vi "Main.vi"() -> ()   [LabVIEW 2020]
uses:
  controls/UI_Ref_Cluster.ctl
  controls/Car_wash_indicators.ctl
  Global variables/Elapsed_time.vi
  Global variables/Time_to_elapse.vi
  Global variables/Bad_position.vi
  Global variables/Delay_time.vi
  Global variables/Reset_timer.vi
  <vilib>/vision/driver/NI_Vision_Acquisition_Software.lvlib
  <vilib>/userDefined/High Color/IMAQdx.ctl
  <vilib>/vision/NI_Vision_Development_Module.lvlib
  <vilib>/drjdpowell/SQLite Library/SQL Connection/Connection.lvclass
  <vilib>/drjdpowell/SQLite Library/SQL Connection/Open (path).vi
  <vilib>/drjdpowell/SQLite Library/SQLite.lvlib
  <vilib>/drjdpowell/SQLite Library/SQL Connection/Execute SQL (No results).vi
  <vilib>/drjdpowell/SQLite Library/SQL Connection/Execute SQL.vi
  controls/Wash_options.ctl
panel:
  out "Result Set":string[][](table) caption="Result Set (from first statement with results)"
  in  "Show Database":bool
  out "SQL_Expression":string
  out "Exit_Panel":bool
  out "Image":T1(plugin-control)
  out "Read String":string
  out "License Plate":string
  in  "Array":i8[](array[numeric])=[0, 1, 2, 3, 4, 5, 6, 7]
  out "Info_for_driver":string
  in  "Car position slider":i8(slide)=1 scale=0.0..7.0
  in  "Start Button":bool
  out "Elapsed Time":dbl format="%.2f"
  in  "Stop Button":bool
  out "Car wash indicators":T2
  in  "Wash Options":T3
  out "Wash entry":bool
  # "Entry console"
  # "Car Wash Dispaly"
  # "Wash Entry"
  # "Wash Options"
  # "Car Wash Indicators"
  # "Car Wash Indicators"
  # "Elapsed Time"
  # "Start"
  # "Car position simulation"
  # "Pre-Soak\nH-P Wash\nL-P Wax\nSpot Free Rinse"
  # "Underbody Wash\nBug Remover"
  # "Tire Shine\nAir Dry"
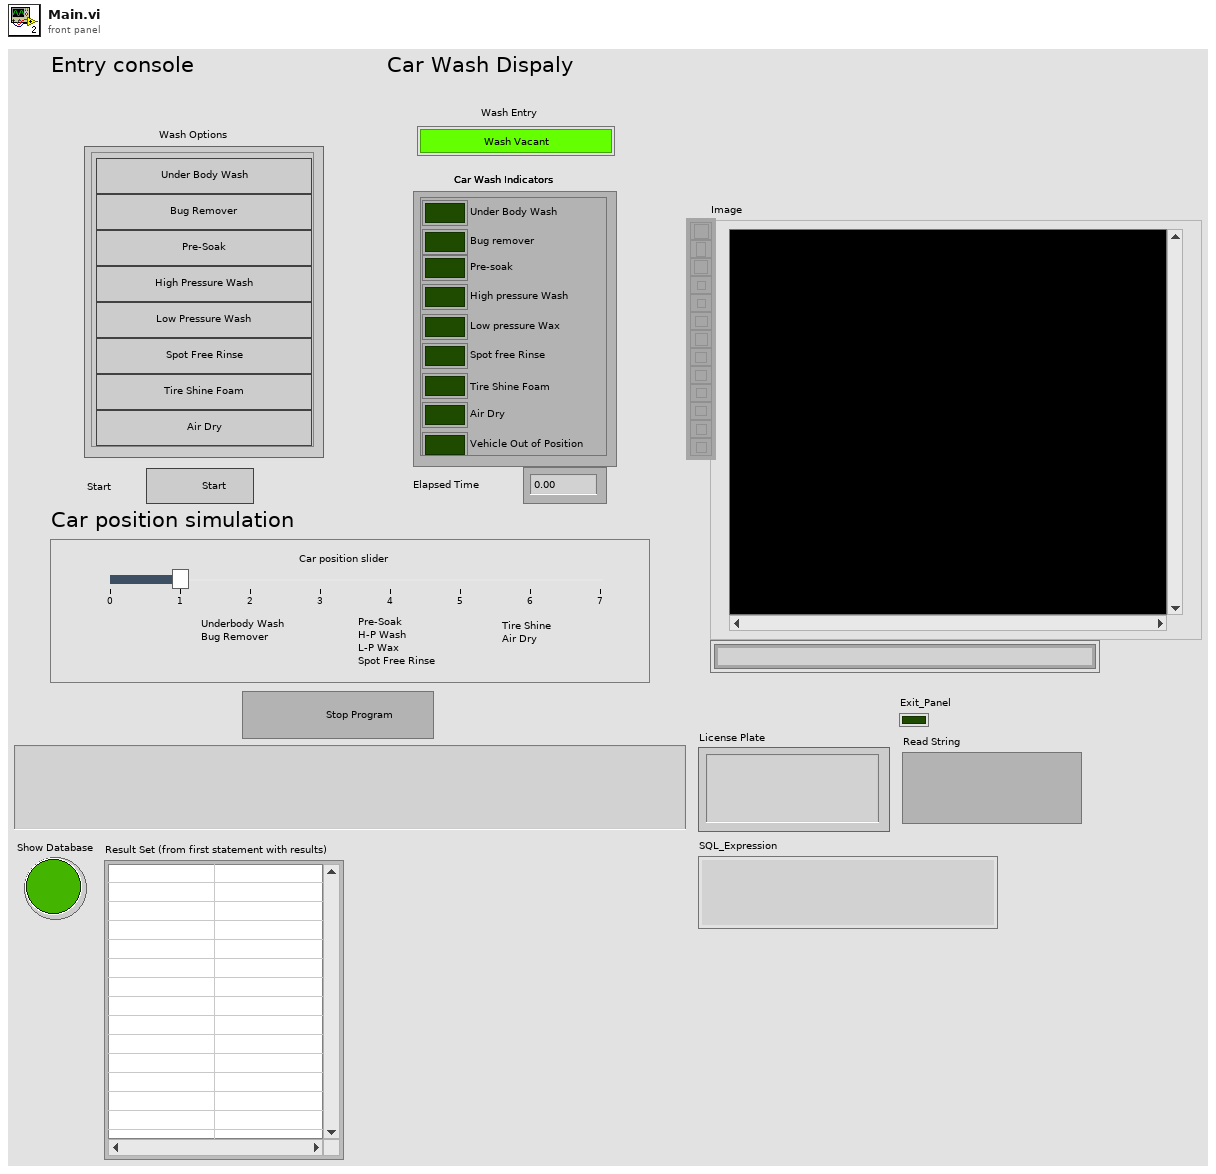
[diagram p1: front panel]
types:
  T1 = typedef "IMAQ Image.ctl" = refnum<image>
  T2 = typedef "Car_wash_indicators.ctl" = cluster{"Under Body Wash":bool, "Bug remover":bool, "Pre-soak":bool, "High pressure Wash":bool, "Low pressure Wax":bool, "Spot free Rinse ":bool, "Tire Shine Foam ":bool, "Air Dry ":bool, "Vehicle Out of Position":bool}
  T3 = typedef "Wash_options.ctl" = cluster{"Under body wash":bool, "Bug remover":bool, "Pre-soak":bool, "High pressure":bool, "Low pressure":bool, "Spot free Rinse":bool, "Tire Shine Foam":bool, "Air Dry":bool}
  T4 = typedef "IMAQ Rectangle" = cluster{"Left":i32, "Top":i32, "Right":i32, "Bottom":i32, "Rotation":dbl}
  T5 = typedef "IMAQdx.ctl" = refnum<k21>
  T6 = typedef "IMAQ OCR Session.ctl" = refnum<k1>
  T7 = enum32{"Invalid", "Standard", "Closed", "Hidden", "Minimized", "Maximized"}
  T8 = enum32{"invalid app kind", "Development System", "Run Time System", "Student Edition", "Embedded LabVIEW", "Evaluation", "Custom"}
  T9 = enum8{"Enabled", "Disabled", "Disabled and Grayed Out"}
  T10 = typedef "UI_Ref_Cluster.ctl" = cluster{"Stop Button Ref":refnum<vi>, "Start Button Ref":refnum<vi>, "Elapsed Time Ref":refnum<vi>, "Car wash indicators Ref":refnum<vi>, "Wash Options Ref":refnum<vi>, "Wash entry Ref":refnum<vi>, "Car position slider Ref":refnum<vi>, "Info_for_driver Ref":refnum<vi>, "Array Ref":refnum<vi>, "License Plate Ref":refnum<vi>}
  T11 = cluster{"Core":cluster{"Current VI Reference":refnum<vi>, "Close Panel on Exit?":bool}, "UI_Cluster_Out":T10}
  T12 = cluster{"Current VI Reference":refnum<vi>, "Close Panel on Exit?":bool}
  T13 = typedef "ROI Descriptor" = cluster{"Global Rectangle":i32[], "Contours":cluster{"ID":enum32{"External", "Internal"}, "Type":u32, "Coordinates":i32[]}[]}
  T14 = cluster{"Global Rectangle":i32[], "Contours":cluster{"ID":enum32{"External", "Internal"}, "Type":u32, "Coordinates":i32[]}[]}
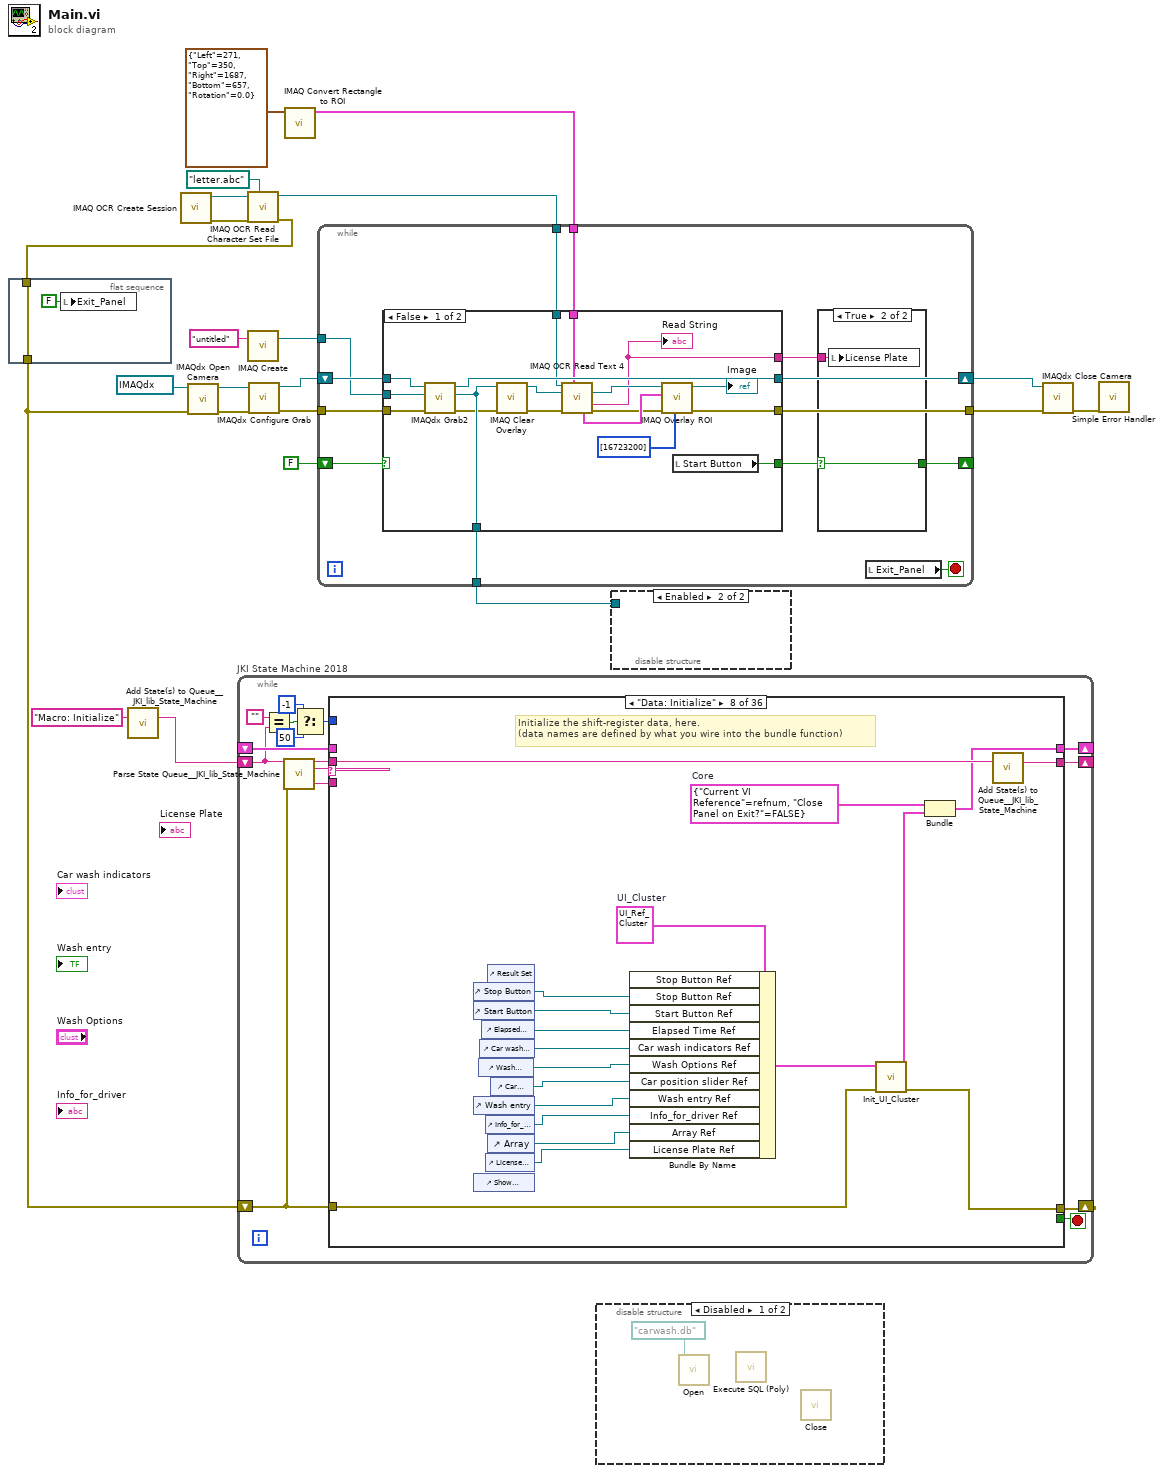
[diagram p0: block diagram]
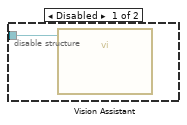
[diagram p2: hidden frame]
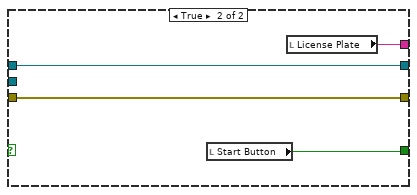
[diagram p5: hidden frame]
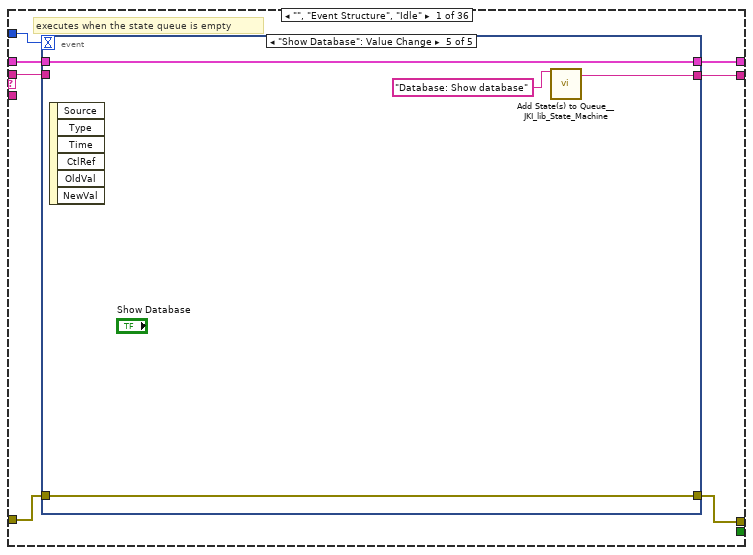
[diagram p6: hidden frame]
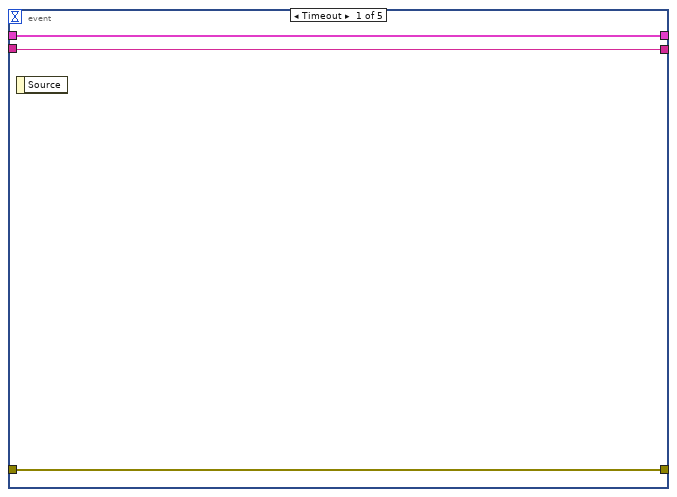
[diagram p7: hidden frame]
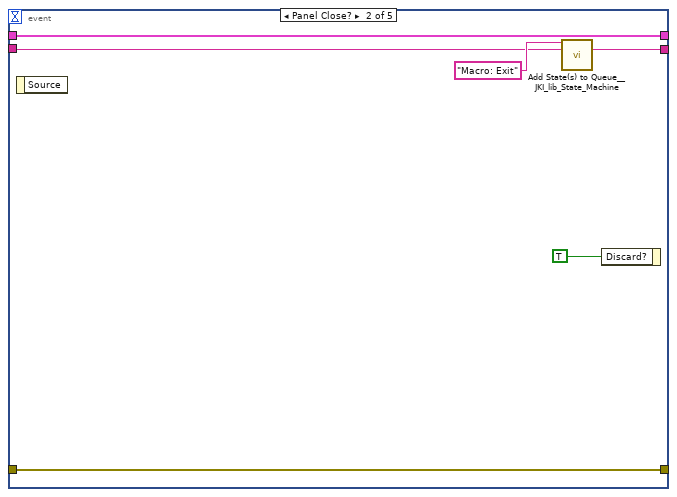
[diagram p8: hidden frame]
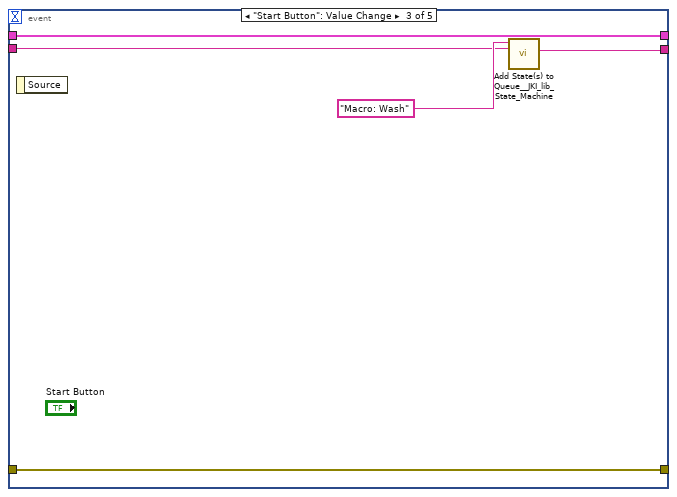
[diagram p9: hidden frame]
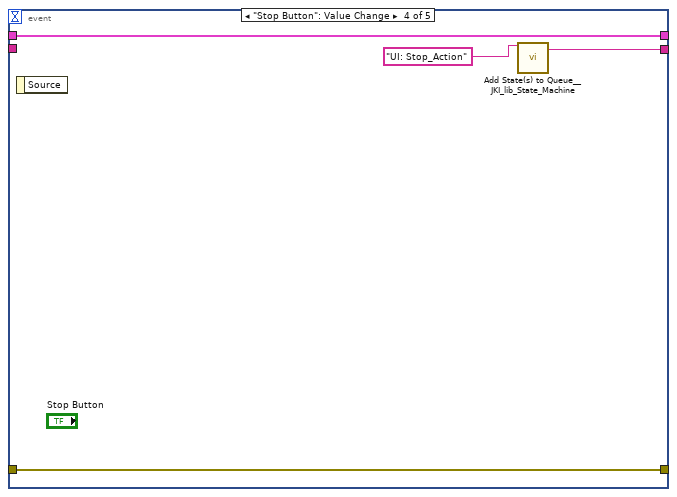
[diagram p10: hidden frame]
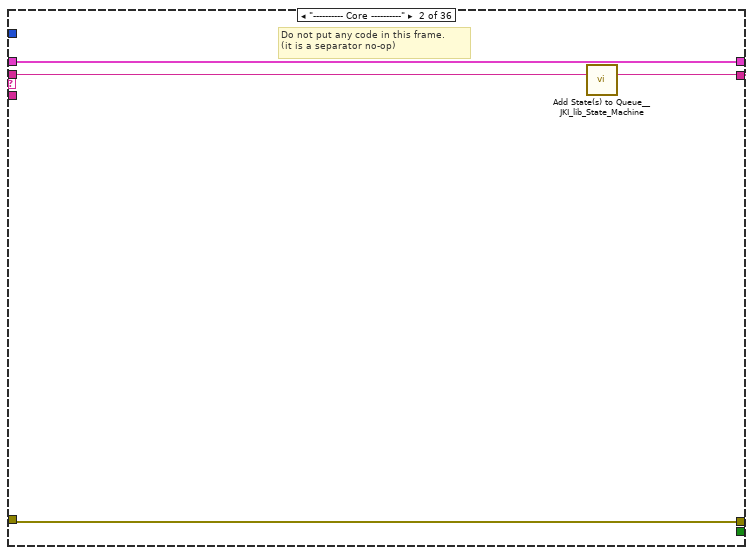
[diagram p11: hidden frame]
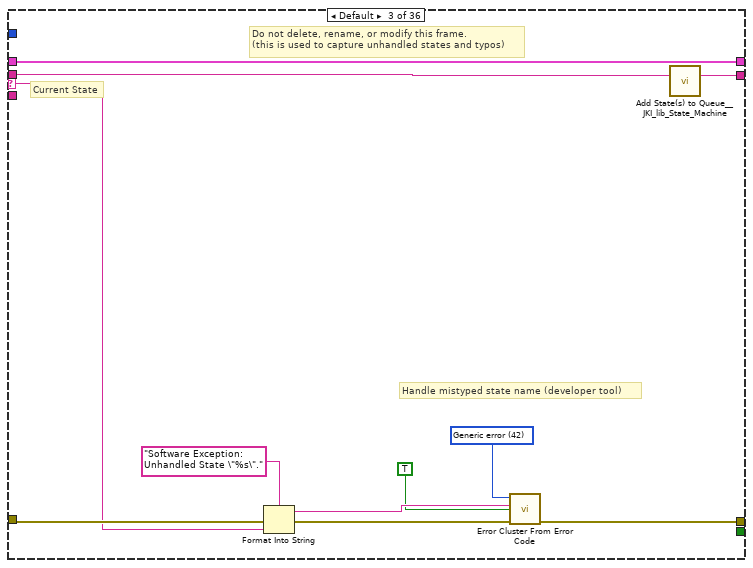
[diagram p12: hidden frame]
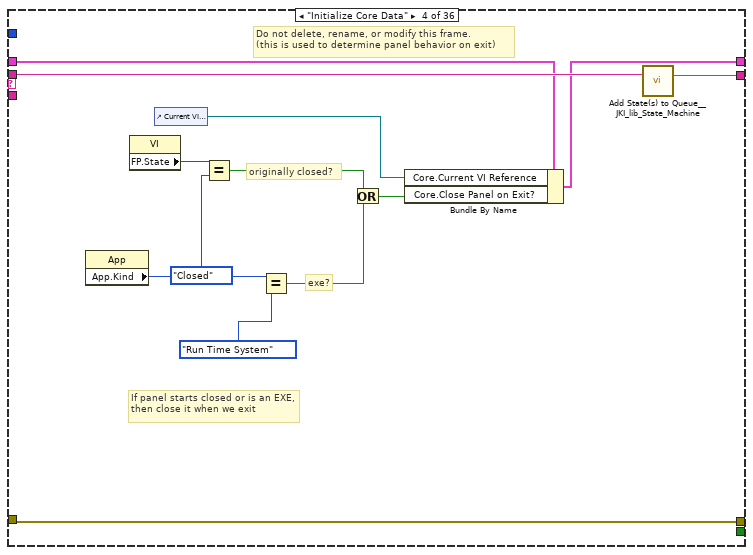
[diagram p13: hidden frame]
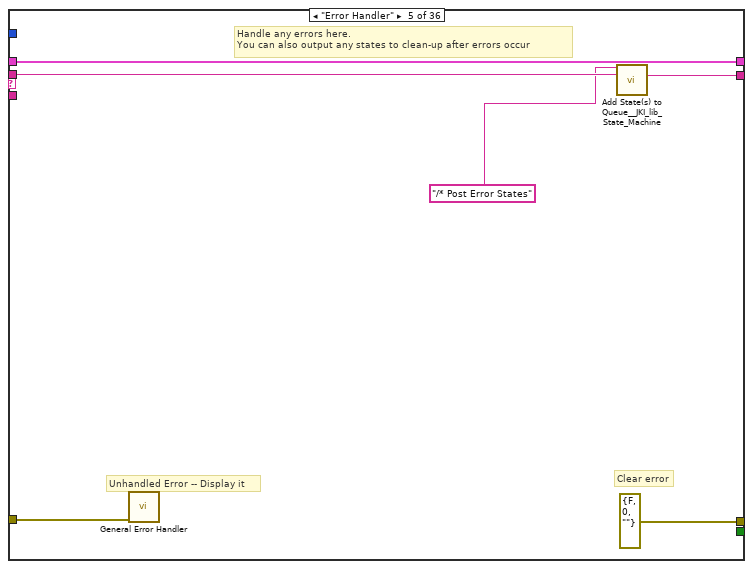
[diagram p14: hidden frame]
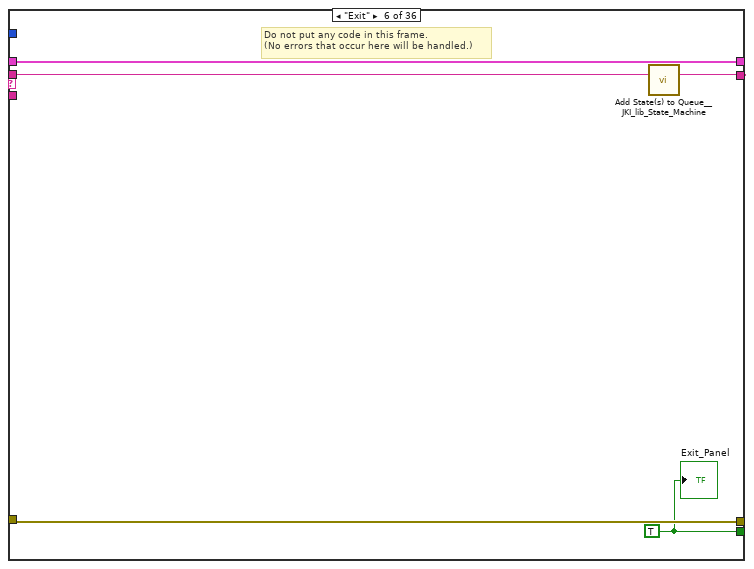
[diagram p15: hidden frame]
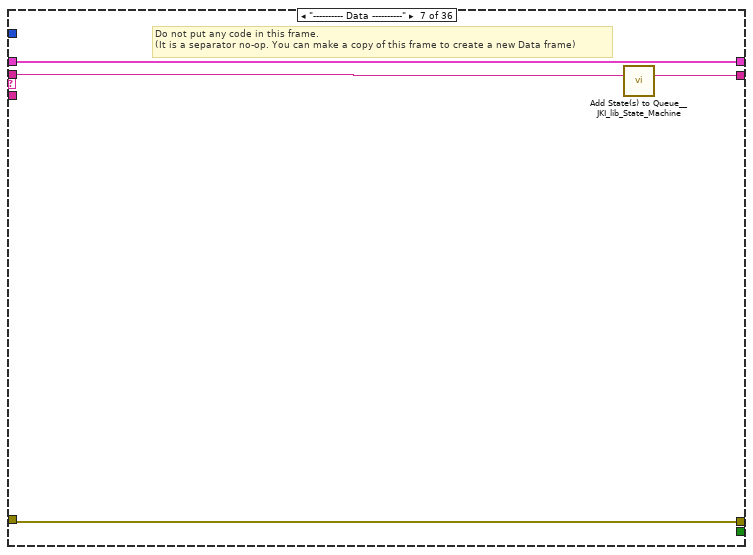
[diagram p16: hidden frame]
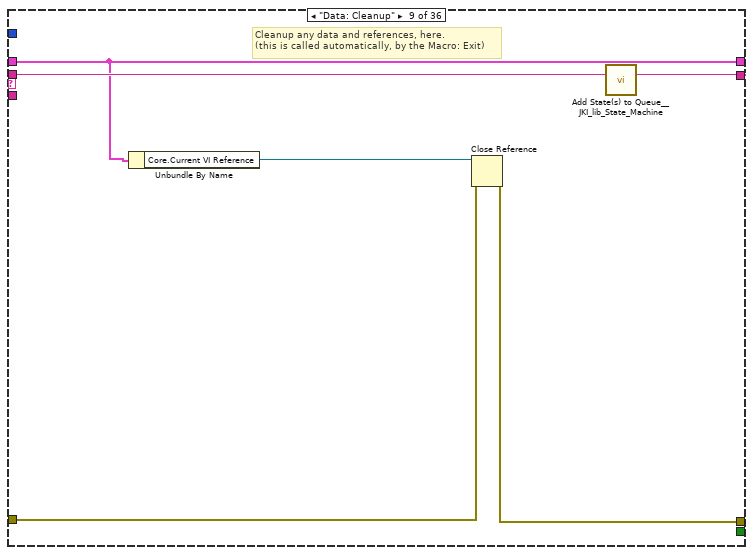
[diagram p17: hidden frame]
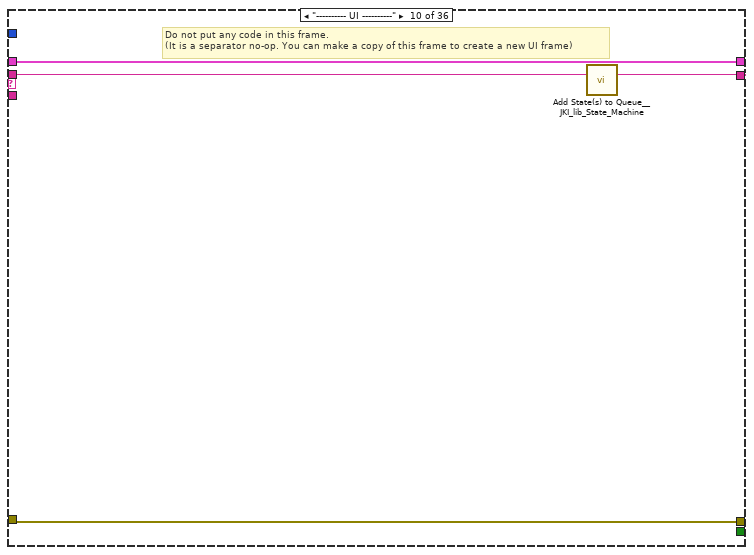
[diagram p18: hidden frame]
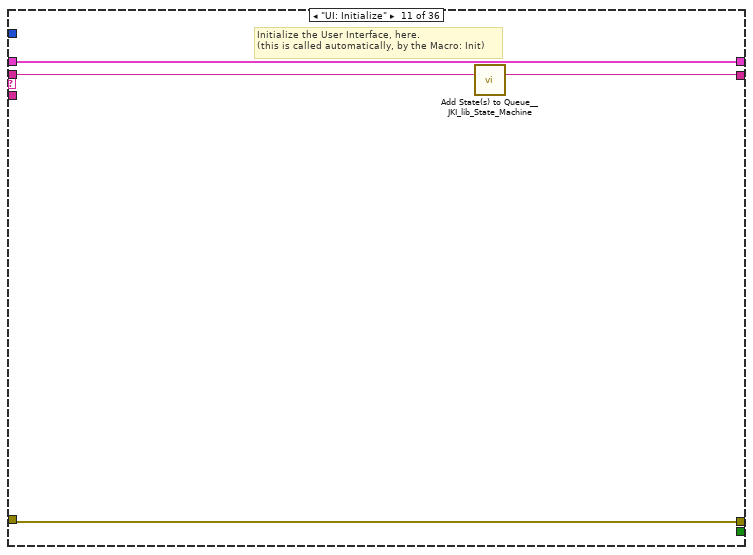
[diagram p19: hidden frame]
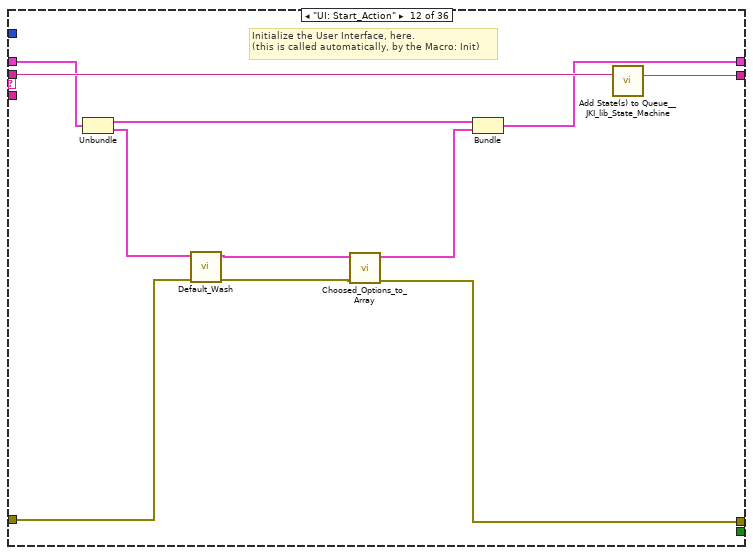
[diagram p20: hidden frame]
diagram:
  n1 = flat-sequence {
    tunnel: w4 -> [w23]
    tunnel: [w23] -> w3
    frame #0 {
      n2 = local write "Exit_Panel"(FALSE) -> ()
    }
  }
  n3 = call <vilib>:"Add State(s) to Queue__JKI_lib_State_Machine.vi"("State(s) in (\"\")"="Macro: Initialize") -> ("States Out"=w22:string)  [unwired: 14 in]
  n4 = call "IMAQ OCR Create Session"() -> ("error out"=w16:errorcluster, "IMAQ OCR Session"=w15:T6)  [unwired: 10 in]
  n5 = call <vilib>:"IMAQdx Open Camera.vi"("error in"=w3, "Session In"=T5 "cam0") -> ("error out"=w7:errorcluster, "Session Out"=w8:T5)  [unwired: 8 in]
  n6 = while "JKI State Machine 2018" {
    shift-right: [w34] -> _
    shift-left: _ -> [w33]
    shift-right: [w36] -> _
    shift-left: w3 -> [w32]
    shift-right: [w35] -> _
    shift-left: w22 -> [w30]
    stop <- w25 stop-if-true
    n7 = Equal?(x="", y=w30) -> (x = y?=w29:bool)
    n8 = call <vilib>:"Parse State Queue__JKI_lib_State_Machine.vi"("State Queue"=w30, "Error In (no error)"=w32) -> ("Remaining States"=w38:string, "Current State"=w39:string, "Arguments"=w37:string)  [unwired: 11 in]
    n9 = Select(t=-1, s=w29, f=50) -> (s? t:f=w28:i32)
    n10 = case shown="\"Data: Initialize\"" w39 {
      selector: w39 -> [_ _ w73 _ _ _ _ _ _ _ _ _ _ _ _ _ _ _ _ _ _ _ _ _ _ _ _ _ _ _ _ _ _ _ _ _]
      tunnel: w38 -> [w41 w72 w77 w96 w102 w107 w111 w130 w136 w140 w144 w155 w164 w170 w181 w245 w250 w255 w265 w269 w273 w303 w306 w339 w379 w419 w459 w499 w539 w579 w619 w658 w664 w671 w684 w689]
      tunnel: w37 -> [_ _ _ _ _ _ _ _ _ _ _ _ _ w166 w176 _ _ _ _ _ _ w300 _ _ _ _ _ _ _ _ _ _ _ _ _ _]
      tunnel: w33 -> [w46 w69 w75 w85 w100 w105 w108 _ w132 w137 w142 w153 w162 w168 w175 w242 w247 w252 w257 w266 w276 w295 w311 w334 w376 w413 w451 w491 w531 w571 w611 w655 w659 w672 w681 w687]
      tunnel: [w45 w70 w79 w94 errorcluster {"status"=FALSE, "code"=0, "source"=""} ("error out") w104 w109 w118 w133 w138 w141 w147 w159 w167 w178 w243 w248 w253 w263 w267 w272 w301 w312 w337 w377 w410 w457 w497 w537 w577 w617 w656 w662 w669 w674 w686] -> w36
      tunnel: w32 -> [w44 w70 w78 w94 w99 w104 w109 w119 w134 w138 w141 w149 w160 w165 w179 w243 w248 w253 w263 w267 w272 w301 w312 w337 w377 w410 w457 w497 w537 w577 w617 w656 w662 w669 w674 w686]
      tunnel: [w40 w71 w76 w95 w101 w106 w110 w129 w135 w139 w143 w154 w163 w169 w180 w244 w249 w254 w264 w268 w277 w302 w305 w338 w378 w418 w458 w498 w538 w578 w618 w657 w663 w670 w683 w688] -> w35
      tunnel: [_ _ _ _ _ w103 _ _ _ _ _ _ _ _ _ _ _ _ _ _ _ _ _ _ _ _ _ _ _ _ _ _ _ _ _ _] -> w25
      tunnel: [w43 w69 w75 w84 w100 w105 w108 w121 w132 w137 w142 w151 w156 w168 w175 w242 w247 w252 w257 w266 w276 w295 w311 w334 w376 w413 w451 w491 w531 w571 w611 w655 w659 w672 w681 w687] -> w34
      tunnel: w28 -> [w42 _ _ _ _ _ _ _ _ _ _ _ _ _ _ _ _ _ _ _ _ _ _ _ _ _ _ _ _ _ _ _ _ _ _ _]
      frame "", "Event Structure", "Idle" {
        # "executes when the state queue is empty"
        n11 = event shown="[4] \"Show Database\": Value Change" {
          selector: _ -> [_ _ _ _ _]
          dyn-events: _ -> [_ _ _ _ _]
          timeout: w42 -> [_ _ _ _ _]
          tunnel: w46 -> [w48 w54 w60 w64 w68]
          tunnel: [w49 w55 w58 w62 w66] -> w45
          tunnel: w44 -> [w49 w55 w58 w62 w66]
          tunnel: [w48 w54 w60 w64 w68] -> w43
          tunnel: [w47 w51 w56 w61 w65] -> w40
          tunnel: w41 -> [w47 w50 w57 _ _]
          event Timeout {
            n12 = event-data() -> ()  [unwired: 1 in, 1 out]
          }
          event Panel Close? {
            n13 = event-data() -> ()  [unwired: 1 in, 1 out]
            n14 = call <vilib>:"Add State(s) to Queue__JKI_lib_State_Machine.vi"("State(s) in Front (\"\")"="Macro: Exit", "State(s) in (\"\")"=w50) -> ("States Out"=w51:string)  [unwired: 13 in]
            n15 = event-data("Discard?"=TRUE) -> ()  [unwired: 1 in, 1 out]
          }
          event "Start Button": Value Change {
            n16 = event-data() -> ()  [unwired: 1 in, 1 out]
            n17 = call <vilib>:"Add State(s) to Queue__JKI_lib_State_Machine.vi"("State(s) in Front (\"\")"="Macro: Wash", "State(s) in (\"\")"=w57) -> ("States Out"=w56:string)  [unwired: 13 in]
          }
          event "Stop Button": Value Change {
            n18 = event-data() -> ()  [unwired: 1 in, 1 out]
            n19 = call <vilib>:"Add State(s) to Queue__JKI_lib_State_Machine.vi"("State(s) in Front (\"\")"="UI: Stop_Action") -> ("States Out"=w61:string)  [unwired: 14 in]
          }
          event "Show Database": Value Change {
            n20 = event-data() -> ()  [unwired: 1 in, 6 out]
            n21 = call <vilib>:"Add State(s) to Queue__JKI_lib_State_Machine.vi"("State(s) in Front (\"\")"="Database: Show database") -> ("States Out"=w65:string)  [unwired: 14 in]
          }
        }
      }
      frame "---------- Core ----------" {
        # "Do not put any code in this frame.\n(it is a separator no-op)"
        n22 = call <vilib>:"Add State(s) to Queue__JKI_lib_State_Machine.vi"("State(s) in (\"\")"=w72) -> ("States Out"=w71:string)  [unwired: 14 in]
      }
      frame Default {
        w82 = 42 items=["No error", "Argument error", "Memory is full", "Out of zone", "End of file", "File already open", "Generic file I/O error", "File not found", "File permission error", "Disk is full", "Duplicate path", "Too many files open", "System feature not enabled", "Resource file not found", "Cannot add resource", "Resource not found", "Image not found", "Image memory error", "Pen does not exist", "Config type invalid", "Config token not found", "Config parse error", "Config memory error", "Bad external code format", "Bad external code offset", "External code not present", "Null window", "Destroy window error", "Null menu", "Print aborted", "Bad print record", "Print driver error", "Windows error during printing", "Memory error during printing", "Print dialog error", "Generic print error", "Invalid device refnum", "Device not found", "Device parameter error", "Device unit error", "Cannot open device", "Device call aborted", "Generic error", "Cancelled by user", "Object ID too low", "Object ID too high", "Object not in heap", "Unknown heap", "Unknown object (invalid DefProc)", "Unknown object (DefProc not in table)", "Message out of range", "Invalid (null) method", "Unknown message", "Manager call not supported", "Bad address", "Network operation in progress", "Network operation timed out", "Connection is busy", "Network attribute not supported", "Network error", "Address in use", "System out of memory", "Connection aborted", "Connection refused", "Not connected", "Already connected", "Connection closed", "Initialization error (interapplication manager)", "Bad occurrence", "Wait on unbound occurrence handler", "Occurrence queue overflow", "Datalog type conflict", "Unused", "Unrecognized type (interapplication manager)", "Memory corrupt", "Failed to make temporary DLL", "Old CIN version", "Drag socket not found", "Failed to load drop-object", "Failed to register OLE object", "Failed to release OLE object", "Format specifier type mismatch", "Unknown format specifier", "Too few format specifiers", "Too many format specifiers", "Scan failed", "Newer CIN version", "Error converting to variant", "Runtime menu error", "Password tampered", "Variant attribute not found", "Incompatible variant data type", "Event data is not available", "Event Store is not present", "Occurrence is not found", "Event Queue is not created", "Event info is not available", "Refnum passed is NULL", "Error retrieving Class GUID", "Error retrieving CoClass GUID", "Error retrieving TypeLib GUID.", "Bad built application magic bytes.", "Specific driver is different from the specific driver associated with the Logical Name.", "There is no session opened to the class driver.", "Max Error", "MAX - Error with config objects", "MAX - Error loading configuration", "MAX - Group not supported"]
        # "Current State"
        # "Do not delete, rename, or modify this frame.\n(this is used to capture unhandled states and typos)"
        # "Handle mistyped state name (developer tool)"
        n23 = Format Into String(format string="Software Exception: Unhandled State \"%s\"." ("message"), error in=w78, w73) -> (resulting string=w81:string, error out=w80:errorcluster)  [unwired: 1 in]
        n24 = call <vilib>:"Error Cluster From Error Code.vi"("show call chain? (False)"=TRUE, "error in (no error)"=w80, "error message (\"\")"=w81, "error code (0)"=w82) -> ("error out"=w79:errorcluster)  [unwired: 5 in]
        n25 = call <vilib>:"Add State(s) to Queue__JKI_lib_State_Machine.vi"("State(s) in (\"\")"=w77) -> ("States Out"=w76:string)  [unwired: 14 in]
      }
      frame "Initialize Core Data" {
        # "Do not delete, rename, or modify this frame.\n(this is used to determine panel behavior on exit)"
        # "originally closed?"
        # "exe?"
        # "If panel starts closed or is an EXE, then close it when we exit"
        n26 = property class="App"() -> ("App.Kind"=w93:T8)  [unwired: 2 in, 2 out]
        n27 = property class="VI"() -> ("FP.State"=w88:T7)  [unwired: 2 in, 2 out]
        n28 = control-ref of="Current VI Reference"() -> (w89:refnum<vi>)
        n29 = Equal?(x=w88, y=T7."Closed" ("Front Panel Window:State")) -> (x = y?=w86:bool)
        n30 = Equal?(x=w93, y=T8."Run Time System" ("Application:Kind")) -> (x = y?=w91:bool)
        n31 = Or(x=w86, y=w91) -> (x .or. y?=w90:bool)
        n32 = Bundle By Name(cluster=w85, "Core.Current VI Reference"=w89, "Core.Close Panel on Exit?"=w90) -> (w84:T11)
        n33 = call <vilib>:"Add State(s) to Queue__JKI_lib_State_Machine.vi"("State(s) in (\"\")"=w96) -> ("States Out"=w95:string)  [unwired: 14 in]
      }
      frame "Error Handler" {
        # "Unhandled Error -- Display it"
        # "Handle any errors here.\nYou can also output any states to clean-up after errors occur"
        # "Clear error"
        n34 = call <vilib>:"General Error Handler.vi"("error in (no error)"=w99) -> ()  [unwired: 10 in, 5 out]
        n35 = call <vilib>:"Add State(s) to Queue__JKI_lib_State_Machine.vi"("State(s) in Front (\"\")"="/* Post Error States", "State(s) in (\"\")"=w102) -> ("States Out"=w101:string)  [unwired: 13 in]
      }
      frame "Exit" {
        w103 = TRUE
        # "Do not put any code in this frame.\n(No errors that occur here will be handled.)"
        n36 = call <vilib>:"Add State(s) to Queue__JKI_lib_State_Machine.vi"("State(s) in (\"\")"=w107) -> ("States Out"=w106:string)  [unwired: 14 in]
        "Exit_Panel" <- w103
      }
      frame "---------- Data ----------" {
        # "Do not put any code in this frame.\n(It is a separator no-op. You can make a copy of this frame to create a new Data frame)"
        n37 = call <vilib>:"Add State(s) to Queue__JKI_lib_State_Machine.vi"("State(s) in (\"\")"=w111) -> ("States Out"=w110:string)  [unwired: 14 in]
      }
      frame "Data: Initialize" {
        w113 = T10 {"Stop Button Ref"=refnum, "Start Button Ref"=refnum, "Elapsed Time Ref"=refnum, "Car wash indicators Ref"=refnum, "Wash Options Ref"=refnum, "Wash entry Ref"=refnum, "Car position slider Ref"=refnum, "Info_for_driver Ref"=refnum, "Array Ref"=refnum, "License Plate Ref"=refnum}  # UI_Cluster
        w128 = T12 {"Current VI Reference"=refnum, "Close Panel on Exit?"=FALSE}  # Core
        # "Initialize the shift-register data, here.\n(data names are defined by what you wire into the bundle function)"
        n38 = control-ref of="Stop Button"() -> (w126:refnum<vi>)
        n39 = control-ref of="Start Button"() -> (w125:refnum<vi>)
        n40 = control-ref of="Wash entry"() -> (w122:refnum<vi>)
        n41 = control-ref of="Show Database"() -> ()  [unwired: 1 out]
        n42 = control-ref of="Wash Options"() -> (w117:refnum<vi>)
        n43 = control-ref of="Car wash indicators"() -> (w123:refnum<vi>)
        n44 = control-ref of="Elapsed Time"() -> (w124:refnum<vi>)
        n45 = control-ref of="Info_for_driver"() -> (w115:refnum<vi>)
        n46 = control-ref of="License Plate"() -> (w112:refnum<vi>)
        n47 = control-ref of="Result Set"() -> ()  [unwired: 1 out]
        n48 = control-ref of="Array"() -> (w114:refnum<vi>)
        n49 = control-ref of="Car position slider"() -> (w116:refnum<vi>)
        n50 = Bundle By Name "Bundle By Name"(cluster=w113, "Stop Button Ref"=w126, "Start Button Ref"=w125, "Elapsed Time Ref"=w124, "Car wash indicators Ref"=w123, "Wash Options Ref"=w117, "Car position slider Ref"=w116, "Wash entry Ref"=w122, "Info_for_driver Ref"=w115, "Array Ref"=w114, "License Plate Ref"=w112) -> (w127:T10)  [unwired: 1 in]
        n51 = call "Init_UI_Cluster.vi"("UI_Cluster_In"=w127, "error in"=w119) -> ("UI_Cluster_Out"=w120:T10, "error out"=w118:errorcluster)  [unwired: 7 in]
        n52 = Bundle("Core"=w128, "UI_Cluster_Out"=w120) -> (w121:T11)  [unwired: 1 in]
        n53 = call <vilib>:"Add State(s) to Queue__JKI_lib_State_Machine.vi"("State(s) in (\"\")"=w130) -> ("States Out"=w129:string)  [unwired: 14 in]
      }
      frame "Data: Cleanup" {
        # "Cleanup any data and references, here.\n(this is called automatically, by the Macro: Exit)"
        n54 = Unbundle By Name(w132) -> ("Core.Current VI Reference"=w131:refnum<vi>)
        n55 = Close Reference(reference=w131, error in (no error)=w134) -> (error out=w133:errorcluster)
        n56 = call <vilib>:"Add State(s) to Queue__JKI_lib_State_Machine.vi"("State(s) in (\"\")"=w136) -> ("States Out"=w135:string)  [unwired: 14 in]
      }
      frame "---------- UI ----------" {
        # "Do not put any code in this frame.\n(It is a separator no-op. You can make a copy of this frame to create a new UI frame)"
        n57 = call <vilib>:"Add State(s) to Queue__JKI_lib_State_Machine.vi"("State(s) in (\"\")"=w140) -> ("States Out"=w139:string)  [unwired: 14 in]
      }
      frame "UI: Initialize" {
        # "Initialize the User Interface, here.\n(this is called automatically, by the Macro: Init)"
        n58 = call <vilib>:"Add State(s) to Queue__JKI_lib_State_Machine.vi"("State(s) in (\"\")"=w144) -> ("States Out"=w143:string)  [unwired: 14 in]
      }
      frame "UI: Start_Action" {
        # "Initialize the User Interface, here.\n(this is called automatically, by the Macro: Init)"
        n59 = Unbundle(w153) -> ("Core"=w152:T12, "UI_Cluster_Out"=w150:T10)
        n60 = call "Default_Wash.vi"("UI_Cluster_In"=w150, "error in"=w149) -> ("UI_Cluster_Out"=w145:T10, "error out"=w148:errorcluster)  [unwired: 7 in]
        n61 = call "Choosed_Options_to_Array.vi"("error in (no error)"=w148, "UI_Cluster_In"=w145) -> ("error out"=w147:errorcluster, "UI_Cluster_Out"=w146:T10)  [unwired: 8 in]
        n62 = Bundle("Core"=w152, "UI_Cluster_Out"=w146) -> (w151:T11)  [unwired: 1 in]
        n63 = call <vilib>:"Add State(s) to Queue__JKI_lib_State_Machine.vi"("State(s) in (\"\")"=w155) -> ("States Out"=w154:string)  [unwired: 14 in]
      }
      frame "UI: Stop_Action" {
        n64 = Unbundle(w162) -> ("Core"=w158:T12, "UI_Cluster_Out"=w161:T10)
        n65 = call "Stop_UI_Cluster.vi"("UI_Cluster_In"=w161, "error in"=w160) -> ("UI_Cluster_Out"=w157:T10, "error out"=w159:errorcluster)  [unwired: 7 in]
        n66 = Bundle("Core"=w158, "UI_Cluster_Out"=w157) -> (w156:T11)  [unwired: 1 in]
        n67 = call <vilib>:"Add State(s) to Queue__JKI_lib_State_Machine.vi"("State(s) in (\"\")"=w164) -> ("States Out"=w163:string)  [unwired: 14 in]
      }
      frame "UI: Cursor Set" {
        # "Argument"
        # "Set and Unset Cursor Busy.\n(Usage: \"UI: Cursor Set >> Busy|Idle\")"
        n68 = case shown="\"Idle\", Default" w166 {
          tunnel: w165 -> [w172 w174]
          tunnel: [w171 w173] -> w167
          frame "Idle", Default {
            n69 = call <vilib>:"Unset Busy.vi"("error in (no error)"=w172) -> ("error out"=w171:errorcluster)  [unwired: 10 in]
          }
          frame "Busy" {
            n70 = call <vilib>:"Set Busy.vi"("error in (no error)"=w174) -> ("error out"=w173:errorcluster)  [unwired: 9 in, 1 out]
          }
        }
        n71 = call <vilib>:"Add State(s) to Queue__JKI_lib_State_Machine.vi"("State(s) in (\"\")"=w170) -> ("States Out"=w169:string)  [unwired: 14 in]
      }
      frame "UI: Front Panel State" {
        # "Argument"
        # "Set Front Panel Open or Closed\n(Usage: \"UI: Front Panel State >> Open|Close\")"
        n72 = Unbundle By Name(w175) -> ("Core.Current VI Reference"=w177:refnum<vi>)
        n73 = case shown="\"Minimize\", \"Minimized\"" w176 {
          tunnel: w179 -> [w187 w200 w211 w223 w235]
          tunnel: [w188 w201 w212 w224 w236] -> w178
          tunnel: w177 -> [_ _ _ _ _]
          frame "Open", "Standard", Default {
            w182 = T7."Standard" ("State")
            n74 = property class="VI"(error in=w187) -> (reference out=w185:refnum<vi>, error out=w186:errorcluster, "FP.State"=w184:T7)  [unwired: 1 in]
            n75 = Not Equal?(x=w184, y=w182) -> (x != y?=w183:bool)
            n76 = case shown="True" w183 {
              tunnel: [w192 w194] -> w188
              tunnel: w186 -> [w191 w194]
              tunnel: w185 -> [w190 _]
              tunnel: w182 -> [w189 _]
              frame True {
                n77 = invoke class="VI" method="FP.Open"(reference=w190, error in=w191, "Activate"=TRUE, "State"=w189) -> (error out=w192:errorcluster)  [unwired: 1 in, 4 out]
              }
              frame False {
              }
            }
          }
          frame "Close", "Closed" {
            n78 = property class="VI"(error in=w200) -> (reference out=w198:refnum<vi>, error out=w199:errorcluster, "FP.State"=w196:T7)  [unwired: 1 in]
            n79 = Not Equal?(x=w196, y=T7."Closed" ("Front Panel Window:State")) -> (x != y?=w195:bool)
            n80 = case shown="True" w195 {
              tunnel: [w202 w205] -> w201
              tunnel: w199 -> [w202 w204]
              tunnel: w198 -> [_ w203]
              frame False {
              }
              frame True {
                n81 = invoke class="VI" method="FP.Close"(reference=w203, error in=w204) -> (error out=w205:errorcluster)  [unwired: 1 in, 2 out]
              }
            }
          }
          frame "Hidden", "Hide" {
            w206 = T7."Hidden" ("State")
            n82 = property class="VI"(error in=w211) -> (reference out=w209:refnum<vi>, error out=w210:errorcluster, "FP.State"=w208:T7)  [unwired: 1 in]
            n83 = Not Equal?(x=w208, y=w206) -> (x != y?=w207:bool)
            n84 = case shown="True" w207 {
              tunnel: [w216 w217] -> w212
              tunnel: w210 -> [w215 w217]
              tunnel: w209 -> [w214 _]
              tunnel: w206 -> [w213 _]
              frame True {
                n85 = invoke class="VI" method="FP.Open"(reference=w214, error in=w215, "State"=w213) -> (error out=w216:errorcluster)  [unwired: 2 in, 4 out]
              }
              frame False {
              }
            }
          }
          frame "Minimize", "Minimized" {
            w218 = T7."Minimized" ("State")
            n86 = property class="VI"(error in=w223) -> (reference out=w221:refnum<vi>, error out=w222:errorcluster, "FP.State"=w220:T7)  [unwired: 1 in]
            n87 = Not Equal?(x=w220, y=w218) -> (x != y?=w219:bool)
            n88 = case shown="True" w219 {
              tunnel: [w228 w229] -> w224
              tunnel: w222 -> [w227 w229]
              tunnel: w221 -> [w226 _]
              tunnel: w218 -> [w225 _]
              frame True {
                n89 = invoke class="VI" method="FP.Open"(reference=w226, error in=w227, "State"=w225) -> (error out=w228:errorcluster)  [unwired: 2 in, 4 out]
              }
              frame False {
              }
            }
          }
          frame "Maximize", "Maximized" {
            w230 = T7."Maximized" ("State")
            n90 = property class="VI"(error in=w235) -> (reference out=w233:refnum<vi>, error out=w234:errorcluster, "FP.State"=w232:T7)  [unwired: 1 in]
            n91 = Not Equal?(x=w232, y=w230) -> (x != y?=w231:bool)
            n92 = case shown="True" w231 {
              tunnel: [w240 w241] -> w236
              tunnel: w234 -> [w239 w241]
              tunnel: w233 -> [w238 _]
              tunnel: w230 -> [w237 _]
              frame True {
                n93 = invoke class="VI" method="FP.Open"(reference=w238, error in=w239, "State"=w237) -> (error out=w240:errorcluster)  [unwired: 2 in, 4 out]
              }
              frame False {
              }
            }
          }
        }
        n94 = call <vilib>:"Add State(s) to Queue__JKI_lib_State_Machine.vi"("State(s) in (\"\")"=w181) -> ("States Out"=w180:string)  [unwired: 14 in]
      }
      frame "---------- Macro ----------" {
        # "Do not put any code in this frame.\n(It is a separator no-op. You can make a copy of this frame to create a new Macro frame)"
        n95 = call <vilib>:"Add State(s) to Queue__JKI_lib_State_Machine.vi"("State(s) in (\"\")"=w245) -> ("States Out"=w244:string)  [unwired: 14 in]
      }
      frame "Macro: Wash" {
        # "Do not put any code in this frame.\n(It is a separator no-op. You can make a copy of this frame to create a new Macro frame)"
        n96 = call <vilib>:"Add State(s) to Queue__JKI_lib_State_Machine.vi"("State(s) in Front (\"\")"="UI: Start_Action\nProgress: Option_choose \nProgress: Reset variables_to leave\nProgress: Wait for slider\nUI: Stop_Action" ("State(s) in Front (\"\")"), "State(s) in (\"\")"=w250) -> ("States Out"=w249:string)  [unwired: 13 in]
      }
      frame "Macro: Initialize" {
        # "Initialization Macro\n(This is called once, when the VI starts)"
        n97 = call <vilib>:"Add State(s) to Queue__JKI_lib_State_Machine.vi"("State(s) in Front (\"\")"="Data: Initialize\nInitialize Core Data\nUI: Initialize\nUI: Front Panel State >> Open", "State(s) in (\"\")"=w255) -> ("States Out"=w254:string)  [unwired: 13 in]
      }
      frame "Macro: Exit" {
        # "Exit Macro\n(This is called once, when the VI exits)"
        n98 = Unbundle By Name(w257) -> ("Core.Close Panel on Exit?"=w256:bool)
        n99 = Select(t="UI: Front Panel State >> Close", s=w256, f="") -> (s? t:f=w260:string)
        n100 = call <vilib>:"Add State(s) to Queue__JKI_lib_State_Machine.vi"("State(s) in (\"\")"=w260, "State(s) at Back (\"\")"="Data: Cleanup\nExit") -> ("States Out"=w258:string)  [unwired: 13 in]
        n101 = call <vilib>:"Add State(s) to Queue__JKI_lib_State_Machine.vi"("State(s) in Front (\"\")"=w258, "State(s) in (\"\")"=w265) -> ("States Out"=w264:string)  [unwired: 13 in]
      }
      frame "--------- Progress ----------" {
        # "Your code here.\n(You can make a copy of, or modify, this frame)"
        n102 = call <vilib>:"Add State(s) to Queue__JKI_lib_State_Machine.vi"("State(s) in (\"\")"=w269) -> ("States Out"=w268:string)  [unwired: 14 in]
      }
      frame "Progress: Option_choose" {
        # "Your code here.\n(You can make a copy of, or modify, this frame)"
        n103 = Array Size(array="Array") -> (size(s)=w275:i32)
        n104 = for {
          N: w275 -> [_]
          tunnel: "Array" -> [w283]
          shift-right: [w279] -> w271
          shift-left: "" -> [w278]
          i -> [w282]
          n105 = Index Array(array=w283, index=w282) -> (element=w281:i8)
          n106 = case shown="Default" w281 {
            tunnel: [_ "Progress: Set_wait_time >> 5\nProgress: Option0\n" ("State(s) in Front (\"\")") "Progress: Set_wait_time >> 5\nProgress: Option1\n" ("State(s) in Front (\"\")") "Progress: Set_wait_time >> 5\nProgress: Option2\n" ("State(s) in Front (\"\")") "Progress: Set_wait_time >> 5\nProgress: Option3\n" ("State(s) in Front (\"\")") "Progress: Set_wait_time >> 5\nProgress: Option4\n" ("State(s) in Front (\"\")") "Progress: Set_wait_time >> 5\nProgress: Option5\n" ("State(s) in Front (\"\")") "Progress: Set_wait_time >> 5\nProgress: Option6\n" ("State(s) in Front (\"\")") "Progress: Set_wait_time >> 5\nProgress: Option7\n" ("State(s) in Front (\"\")")] -> w280
            frame Default {
            }
            frame 0 {
            }
            frame 1 {
            }
            frame 2 {
            }
            frame 3 {
            }
            frame 4 {
            }
            frame 5 {
            }
            frame 6 {
            }
            frame 7 {
            }
          }
          n107 = Concatenate Strings(w278, w280) -> (w279:string)
        }
        n108 = call <vilib>:"Add State(s) to Queue__JKI_lib_State_Machine.vi"("State(s) in Front (\"\")"=w271, "State(s) in (\"\")"=w273) -> ("States Out"=w277:string)  [unwired: 13 in]
      }
      frame "Progress: Set_wait_time" {
        w293 = T2 {"Under Body Wash"=FALSE, "Bug remover"=FALSE, "Pre-soak"=FALSE, "High pressure Wash"=FALSE, "Low pressure Wax"=FALSE, "Spot free Rinse "=FALSE, "Tire Shine Foam "=FALSE, "Air Dry "=FALSE, "Vehicle Out of Position"=FALSE}  # Car wash indicators
        # "Your code here.\n(You can make a copy of, or modify, this frame)"
        n109 = Decimal String To Number(string=w300) -> (number=w299:i32)  [unwired: 2 in, 1 out]
        n110 = global write "Elapsed_time.vi" "Numeric"(0.0 ("Numeric")) -> ()
        n111 = global write "Delay_time.vi" "Numeric"(0.0 ("Numeric")) -> ()
        n112 = global write "Reset_timer.vi" "Boolean"(TRUE ("Boolean")) -> ()
        n113 = global write "Bad_position.vi" "Boolean"(FALSE ("Boolean")) -> ()
        n114 = global write "Time_to_elapse.vi" "Numeric"(w299) -> ()
        n115 = Unbundle By Name(w295) -> ("UI_Cluster_Out.Car wash indicators Ref"=w294:refnum<vi>)
        n116 = property class="Clust"(reference=w294, "Value"=w293) -> ()  [unwired: 1 in, 2 out]
        n117 = call <vilib>:"Add State(s) to Queue__JKI_lib_State_Machine.vi"("State(s) in (\"\")"=w303) -> ("States Out"=w302:string)  [unwired: 14 in]
      }
      frame "Progress: Timer" {
        # "Your code here.\n(You can make a copy of, or modify, this frame)"
        n118 = global read "Reset_timer.vi" "Boolean"() -> (w304:bool)
        n119 = flat-sequence {
          tunnel: w310 -> [w318]
          tunnel: w310 -> [w326]
          tunnel: [w327] -> w308
          frame #0 {
            n120 = global read "Bad_position.vi" "Boolean"() -> (w319:bool)
            n121 = case shown="True" w319 {
              tunnel: w318 -> [_ w324]
              frame False {
              }
              frame True {
                n122 = global read "Delay_time.vi" "Numeric"() -> (w321:dbl)
                n123 = global read "Elapsed_time.vi" "Numeric"() -> (w323:dbl)
                n124 = global write "Bad_position.vi" "Boolean"(FALSE ("Boolean")) -> ()
                n125 = Subtract(x=w324, y=w323) -> (x-y=w322:dbl)
                n126 = Add(x=w322, y=w321) -> (x+y=w320:dbl)
                n127 = global write "Delay_time.vi" "Numeric"(w320) -> ()
              }
            }
          }
          frame #1 {
            n128 = global read "Delay_time.vi" "Numeric"() -> (w328:dbl)
            n129 = global write "Elapsed_time.vi" "Numeric"(w326) -> ()
            n130 = Subtract(x=w326, y=w328) -> (x-y=w327:dbl)
            "Elapsed Time" <- w327
          }
          frame #2 {
            n131 = global write "Reset_timer.vi" "Boolean"(FALSE ("Boolean")) -> ()
          }
        }
        n132 = call "Elapsed Time10"("Reset"=w304) -> ("Elapsed Time (s)"=w310:dbl)  [unwired: 11 in, 7 out]
        n133 = global read "Time_to_elapse.vi" "Numeric"() -> (w309:dbl)
        n134 = Less Or Equal?(x=w309, y=w308) -> (x <= y?=w307:bool)
        n135 = case shown="True" w307 {
          tunnel: w306 -> [w314 w317]
          tunnel: [w313 w316] -> w305
          frame False {
            n136 = call <vilib>:"Add State(s) to Queue__JKI_lib_State_Machine.vi"("State(s) in (\"\")"=w314) -> ("States Out"=w313:string)  [unwired: 14 in]
          }
          frame True {
            n137 = local write "Elapsed Time"(0.0 ("Elapsed Time")) -> ()
            n138 = call <vilib>:"Parse State Queue__JKI_lib_State_Machine.vi"("State Queue"=w317) -> ("Remaining States"=w316:string)  [unwired: 12 in, 2 out]
          }
        }
      }
      frame "Progress: Option0" {
        # "Your code here.\n(You can make a copy of, or modify, this frame)"
        n139 = Unbundle By Name(w334) -> ("UI_Cluster_Out"=w333:T10)
        n140 = Unbundle By Name(w333) -> ("Car position slider Ref"=w332:refnum<vi>, "Info_for_driver Ref"=w331:refnum<vi>, "Car wash indicators Ref"=w330:refnum<vi>)
        n141 = property class="Slide (strict)"(reference=w332) -> ("Value"=w336:i8)  [unwired: 1 in, 2 out]
        n142 = case shown="0, Default" w336 {
          tunnel: w331 -> [w341 _]
          tunnel: [w342 "Idle\nProgress: Timer \nProgress: Option0\n " ("State(s) in Front (\"\")")] -> w335
          tunnel: w330 -> [w340 w360]
          frame 0, Default {
            n143 = global read "Bad_position.vi" "Boolean"() -> (w343:bool)
            n144 = case shown="True" w343 {
              tunnel: w341 -> [w347 _]
              tunnel: ["Idle\nProgress: Option0" ("State(s) in Front (\"\")") "Idle\nProgress: Option0" ("State(s) in Front (\"\")")] -> w342
              tunnel: w340 -> [w344 _]
              frame False {
                n145 = property class="Clust"(reference=w344) -> ("Controls[]"=w345:refnum<vi>[])  [unwired: 1 in, 2 out]
                n146 = Index Array(array=w345, index #1=0 ("index"), index #2=8 ("index")) -> (element #1=w351:refnum<vi>, element #2=w349:refnum<vi>)
                n147 = property class="Str"(reference=w347, "Value"="JedŸ do stacji 1") -> ()  [unwired: 1 in, 2 out]
                n148 = global write "Bad_position.vi" "Boolean"(TRUE ("Boolean")) -> ()
                n149 = To Variant(anything=FALSE) -> (Variant=w352:variant)
                n150 = To Variant(anything=TRUE) -> (Variant=w356:variant)
                n151 = property class="Ctl"(reference=w351, "Value"=w352) -> ()  [unwired: 1 in, 2 out]
                n152 = property class="Ctl"(reference=w349, "Value"=w356) -> ()  [unwired: 1 in, 2 out]
              }
              frame True {
              }
            }
          }
          frame 2 {
            n153 = property class="Clust"(reference=w360) -> ("Controls[]"=w359:refnum<vi>[])  [unwired: 1 in, 2 out]
            n154 = Index Array(array=w359, index #1=0 ("index"), index #2=8 ("index")) -> (element #1=w366:refnum<vi>, element #2=w362:refnum<vi>)
            n155 = To Variant(anything=TRUE) -> (Variant=w365:variant)
            n156 = To Variant(anything=FALSE) -> (Variant=w369:variant)
            n157 = property class="Ctl"(reference=w366, "Value"=w365) -> ()  [unwired: 1 in, 2 out]
            n158 = property class="Ctl"(reference=w362, "Value"=w369) -> ()  [unwired: 1 in, 2 out]
          }
        }
        n159 = call <vilib>:"Add State(s) to Queue__JKI_lib_State_Machine.vi"("State(s) in Front (\"\")"=w335, "State(s) in (\"\")"=w339) -> ("States Out"=w338:string)  [unwired: 13 in]
      }
      frame "Progress: Option1" {
        # "Your code here.\n(You can make a copy of, or modify, this frame)"
        n160 = Unbundle By Name(w376) -> ("UI_Cluster_Out"=w374:T10)
        n161 = Unbundle By Name(w374) -> ("Car position slider Ref"=w375:refnum<vi>, "Info_for_driver Ref"=w372:refnum<vi>, "Car wash indicators Ref"=w370:refnum<vi>)
        n162 = property class="Slide (strict)"(reference=w375) -> ("Value"=w373:i8)  [unwired: 1 in, 2 out]
        n163 = case shown="2" w373 {
          tunnel: w372 -> [w381 _]
          tunnel: [w382 "Idle\nProgress: Timer \nProgress: Option1\n " ("State(s) in Front (\"\")")] -> w371
          tunnel: w370 -> [w380 w399]
          frame 0, Default {
            n164 = global read "Bad_position.vi" "Boolean"() -> (w383:bool)
            n165 = case shown="False" w383 {
              tunnel: w381 -> [w387 _]
              tunnel: ["Idle\nProgress: Option1" ("State(s) in Front (\"\")") "Idle\nProgress: Option1" ("State(s) in Front (\"\")")] -> w382
              tunnel: w380 -> [w384 _]
              frame False {
                n166 = property class="Clust"(reference=w384) -> ("Controls[]"=w385:refnum<vi>[])  [unwired: 1 in, 2 out]
                n167 = Index Array(array=w385, index #1=1 ("index"), index #2=8 ("index")) -> (element #1=w391:refnum<vi>, element #2=w389:refnum<vi>)
                n168 = property class="Str"(reference=w387, "Value"="JedŸ do stacji 1") -> ()  [unwired: 1 in, 2 out]
                n169 = global write "Bad_position.vi" "Boolean"(TRUE ("Boolean")) -> ()
                n170 = To Variant(anything=FALSE) -> (Variant=w392:variant)
                n171 = To Variant(anything=TRUE) -> (Variant=w396:variant)
                n172 = property class="Ctl"(reference=w391, "Value"=w392) -> ()  [unwired: 1 in, 2 out]
                n173 = property class="Ctl"(reference=w389, "Value"=w396) -> ()  [unwired: 1 in, 2 out]
              }
              frame True {
              }
            }
          }
          frame 2 {
            n174 = property class="Clust"(reference=w399) -> ("Controls[]"=w400:refnum<vi>[])  [unwired: 1 in, 2 out]
            n175 = Index Array(array=w400, index #1=1 ("index"), index #2=8 ("index")) -> (element #1=w406:refnum<vi>, element #2=w402:refnum<vi>)
            n176 = To Variant(anything=TRUE) -> (Variant=w405:variant)
            n177 = To Variant(anything=FALSE) -> (Variant=w409:variant)
            n178 = property class="Ctl"(reference=w406, "Value"=w405) -> ()  [unwired: 1 in, 2 out]
            n179 = property class="Ctl"(reference=w402, "Value"=w409) -> ()  [unwired: 1 in, 2 out]
          }
        }
        n180 = call <vilib>:"Add State(s) to Queue__JKI_lib_State_Machine.vi"("State(s) in Front (\"\")"=w371, "State(s) in (\"\")"=w379) -> ("States Out"=w378:string)  [unwired: 13 in]
      }
      frame "Progress: Option2" {
        # "Your code here.\n(You can make a copy of, or modify, this frame)"
        n181 = Unbundle By Name(w413) -> ("UI_Cluster_Out"=w412:T10)
        n182 = Unbundle By Name(w412) -> ("Car position slider Ref"=w417:refnum<vi>, "Info_for_driver Ref"=w415:refnum<vi>, "Car wash indicators Ref"=w414:refnum<vi>)
        n183 = property class="Slide (strict)"(reference=w417) -> ("Value"=w416:i8)  [unwired: 1 in, 2 out]
        n184 = case shown="4" w416 {
          tunnel: w415 -> [w421 _]
          tunnel: [w422 "Idle\nProgress: Timer \nProgress: Option2\n " ("State(s) in Front (\"\")")] -> w411
          tunnel: w414 -> [w420 w439]
          frame 0, Default {
            n185 = global read "Bad_position.vi" "Boolean"() -> (w423:bool)
            n186 = case shown="False" w423 {
              tunnel: w421 -> [w427 _]
              tunnel: ["Idle\nProgress: Option2" ("State(s) in Front (\"\")") "Idle\nProgress: Option2" ("State(s) in Front (\"\")")] -> w422
              tunnel: w420 -> [w424 _]
              frame False {
                n187 = property class="Clust"(reference=w424) -> ("Controls[]"=w425:refnum<vi>[])  [unwired: 1 in, 2 out]
                n188 = Index Array(array=w425, index #1=2 ("index"), index #2=8 ("index")) -> (element #1=w431:refnum<vi>, element #2=w429:refnum<vi>)
                n189 = property class="Str"(reference=w427, "Value"="JedŸ do stacji 2") -> ()  [unwired: 1 in, 2 out]
                n190 = global write "Bad_position.vi" "Boolean"(TRUE ("Boolean")) -> ()
                n191 = To Variant(anything=FALSE) -> (Variant=w432:variant)
                n192 = To Variant(anything=TRUE) -> (Variant=w436:variant)
                n193 = property class="Ctl"(reference=w431, "Value"=w432) -> ()  [unwired: 1 in, 2 out]
                n194 = property class="Ctl"(reference=w429, "Value"=w436) -> ()  [unwired: 1 in, 2 out]
              }
              frame True {
              }
            }
          }
          frame 4 {
            n195 = property class="Clust"(reference=w439) -> ("Controls[]"=w440:refnum<vi>[])  [unwired: 1 in, 2 out]
            n196 = Index Array(array=w440, index #1=2 ("index"), index #2=8 ("index")) -> (element #1=w446:refnum<vi>, element #2=w442:refnum<vi>)
            n197 = To Variant(anything=TRUE) -> (Variant=w445:variant)
            n198 = To Variant(anything=FALSE) -> (Variant=w449:variant)
            n199 = property class="Ctl"(reference=w446, "Value"=w445) -> ()  [unwired: 1 in, 2 out]
            n200 = property class="Ctl"(reference=w442, "Value"=w449) -> ()  [unwired: 1 in, 2 out]
          }
        }
        n201 = call <vilib>:"Add State(s) to Queue__JKI_lib_State_Machine.vi"("State(s) in Front (\"\")"=w411, "State(s) in (\"\")"=w419) -> ("States Out"=w418:string)  [unwired: 13 in]
      }
      frame "Progress: Option3" {
        # "Your code here.\n(You can make a copy of, or modify, this frame)"
        n202 = Unbundle By Name(w451) -> ("UI_Cluster_Out"=w452:T10)
        n203 = Unbundle By Name(w452) -> ("Car position slider Ref"=w456:refnum<vi>, "Info_for_driver Ref"=w454:refnum<vi>, "Car wash indicators Ref"=w453:refnum<vi>)
        n204 = property class="Slide (strict)"(reference=w456) -> ("Value"=w455:i8)  [unwired: 1 in, 2 out]
        n205 = case shown="4" w455 {
          tunnel: w454 -> [w461 _]
          tunnel: [w462 "Idle\nProgress: Timer \nProgress: Option3\n " ("State(s) in Front (\"\")")] -> w450
          tunnel: w453 -> [w460 w479]
          frame 0, Default {
            n206 = global read "Bad_position.vi" "Boolean"() -> (w463:bool)
            n207 = case shown="True" w463 {
              tunnel: w461 -> [w467 _]
              tunnel: ["Idle\nProgress: Option3" ("State(s) in Front (\"\")") "Idle\nProgress: Option3" ("State(s) in Front (\"\")")] -> w462
              tunnel: w460 -> [w464 _]
              frame False {
                n208 = property class="Clust"(reference=w464) -> ("Controls[]"=w465:refnum<vi>[])  [unwired: 1 in, 2 out]
                n209 = Index Array(array=w465, index #1=3 ("index"), index #2=8 ("index")) -> (element #1=w471:refnum<vi>, element #2=w469:refnum<vi>)
                n210 = property class="Str"(reference=w467, "Value"="JedŸ do stacji 2") -> ()  [unwired: 1 in, 2 out]
                n211 = global write "Bad_position.vi" "Boolean"(TRUE ("Boolean")) -> ()
                n212 = To Variant(anything=FALSE) -> (Variant=w472:variant)
                n213 = To Variant(anything=TRUE) -> (Variant=w476:variant)
                n214 = property class="Ctl"(reference=w471, "Value"=w472) -> ()  [unwired: 1 in, 2 out]
                n215 = property class="Ctl"(reference=w469, "Value"=w476) -> ()  [unwired: 1 in, 2 out]
              }
              frame True {
              }
            }
          }
          frame 4 {
            n216 = property class="Clust"(reference=w479) -> ("Controls[]"=w480:refnum<vi>[])  [unwired: 1 in, 2 out]
            n217 = Index Array(array=w480, index #1=3 ("index"), index #2=8 ("index")) -> (element #1=w486:refnum<vi>, element #2=w482:refnum<vi>)
            n218 = To Variant(anything=TRUE) -> (Variant=w485:variant)
            n219 = To Variant(anything=FALSE) -> (Variant=w489:variant)
            n220 = property class="Ctl"(reference=w486, "Value"=w485) -> ()  [unwired: 1 in, 2 out]
            n221 = property class="Ctl"(reference=w482, "Value"=w489) -> ()  [unwired: 1 in, 2 out]
          }
        }
        n222 = call <vilib>:"Add State(s) to Queue__JKI_lib_State_Machine.vi"("State(s) in Front (\"\")"=w450, "State(s) in (\"\")"=w459) -> ("States Out"=w458:string)  [unwired: 13 in]
      }
      frame "Progress: Option4" {
        # "Your code here.\n(You can make a copy of, or modify, this frame)"
        n223 = Unbundle By Name(w491) -> ("UI_Cluster_Out"=w492:T10)
        n224 = Unbundle By Name(w492) -> ("Car position slider Ref"=w496:refnum<vi>, "Info_for_driver Ref"=w494:refnum<vi>, "Car wash indicators Ref"=w493:refnum<vi>)
        n225 = property class="Slide (strict)"(reference=w496) -> ("Value"=w495:i8)  [unwired: 1 in, 2 out]
        n226 = case shown="4" w495 {
          tunnel: w494 -> [w501 _]
          tunnel: [w502 "Idle\nProgress: Timer \nProgress: Option4\n " ("State(s) in Front (\"\")")] -> w490
          tunnel: w493 -> [w500 w519]
          frame 0, Default {
            n227 = global read "Bad_position.vi" "Boolean"() -> (w503:bool)
            n228 = case shown="False" w503 {
              tunnel: w501 -> [w507 _]
              tunnel: ["Idle\nProgress: Option4" ("State(s) in Front (\"\")") "Idle\nProgress: Option4" ("State(s) in Front (\"\")")] -> w502
              tunnel: w500 -> [w504 _]
              frame False {
                n229 = property class="Clust"(reference=w504) -> ("Controls[]"=w505:refnum<vi>[])  [unwired: 1 in, 2 out]
                n230 = Index Array(array=w505, index #1=4 ("index"), index #2=8 ("index")) -> (element #1=w511:refnum<vi>, element #2=w509:refnum<vi>)
                n231 = property class="Str"(reference=w507, "Value"="JedŸ do stacji 2") -> ()  [unwired: 1 in, 2 out]
                n232 = global write "Bad_position.vi" "Boolean"(TRUE ("Boolean")) -> ()
                n233 = To Variant(anything=FALSE) -> (Variant=w512:variant)
                n234 = To Variant(anything=TRUE) -> (Variant=w516:variant)
                n235 = property class="Ctl"(reference=w511, "Value"=w512) -> ()  [unwired: 1 in, 2 out]
                n236 = property class="Ctl"(reference=w509, "Value"=w516) -> ()  [unwired: 1 in, 2 out]
              }
              frame True {
              }
            }
          }
          frame 4 {
            n237 = property class="Clust"(reference=w519) -> ("Controls[]"=w520:refnum<vi>[])  [unwired: 1 in, 2 out]
            n238 = Index Array(array=w520, index #1=4 ("index"), index #2=8 ("index")) -> (element #1=w526:refnum<vi>, element #2=w522:refnum<vi>)
            n239 = To Variant(anything=TRUE) -> (Variant=w525:variant)
            n240 = To Variant(anything=FALSE) -> (Variant=w529:variant)
            n241 = property class="Ctl"(reference=w526, "Value"=w525) -> ()  [unwired: 1 in, 2 out]
            n242 = property class="Ctl"(reference=w522, "Value"=w529) -> ()  [unwired: 1 in, 2 out]
          }
        }
        n243 = call <vilib>:"Add State(s) to Queue__JKI_lib_State_Machine.vi"("State(s) in Front (\"\")"=w490, "State(s) in (\"\")"=w499) -> ("States Out"=w498:string)  [unwired: 13 in]
      }
      frame "Progress: Option5" {
        # "Your code here.\n(You can make a copy of, or modify, this frame)"
        n244 = Unbundle By Name(w531) -> ("UI_Cluster_Out"=w532:T10)
        n245 = Unbundle By Name(w532) -> ("Car position slider Ref"=w536:refnum<vi>, "Info_for_driver Ref"=w534:refnum<vi>, "Car wash indicators Ref"=w533:refnum<vi>)
        n246 = property class="Slide (strict)"(reference=w536) -> ("Value"=w535:i8)  [unwired: 1 in, 2 out]
        n247 = case shown="4" w535 {
          tunnel: w534 -> [w541 _]
          tunnel: [w542 "Idle\nProgress: Timer \nProgress: Option5\n " ("State(s) in Front (\"\")")] -> w530
          tunnel: w533 -> [w540 w559]
          frame 0, Default {
            n248 = global read "Bad_position.vi" "Boolean"() -> (w543:bool)
            n249 = case shown="False" w543 {
              tunnel: w541 -> [w547 _]
              tunnel: ["Idle\nProgress: Option5" ("State(s) in Front (\"\")") "Idle\nProgress: Option5" ("State(s) in Front (\"\")")] -> w542
              tunnel: w540 -> [w544 _]
              frame False {
                n250 = property class="Clust"(reference=w544) -> ("Controls[]"=w545:refnum<vi>[])  [unwired: 1 in, 2 out]
                n251 = Index Array(array=w545, index #1=5 ("index"), index #2=8 ("index")) -> (element #1=w551:refnum<vi>, element #2=w549:refnum<vi>)
                n252 = property class="Str"(reference=w547, "Value"="JedŸ do stacji 2") -> ()  [unwired: 1 in, 2 out]
                n253 = global write "Bad_position.vi" "Boolean"(TRUE ("Boolean")) -> ()
                n254 = To Variant(anything=FALSE) -> (Variant=w552:variant)
                n255 = To Variant(anything=TRUE) -> (Variant=w556:variant)
                n256 = property class="Ctl"(reference=w551, "Value"=w552) -> ()  [unwired: 1 in, 2 out]
                n257 = property class="Ctl"(reference=w549, "Value"=w556) -> ()  [unwired: 1 in, 2 out]
              }
              frame True {
              }
            }
          }
          frame 4 {
            n258 = property class="Clust"(reference=w559) -> ("Controls[]"=w560:refnum<vi>[])  [unwired: 1 in, 2 out]
            n259 = Index Array(array=w560, index #1=5 ("index"), index #2=8 ("index")) -> (element #1=w566:refnum<vi>, element #2=w562:refnum<vi>)
            n260 = To Variant(anything=TRUE) -> (Variant=w565:variant)
            n261 = To Variant(anything=FALSE) -> (Variant=w569:variant)
            n262 = property class="Ctl"(reference=w566, "Value"=w565) -> ()  [unwired: 1 in, 2 out]
            n263 = property class="Ctl"(reference=w562, "Value"=w569) -> ()  [unwired: 1 in, 2 out]
          }
        }
        n264 = call <vilib>:"Add State(s) to Queue__JKI_lib_State_Machine.vi"("State(s) in Front (\"\")"=w530, "State(s) in (\"\")"=w539) -> ("States Out"=w538:string)  [unwired: 13 in]
      }
      frame "Progress: Option6" {
        # "Your code here.\n(You can make a copy of, or modify, this frame)"
        n265 = Unbundle By Name(w571) -> ("UI_Cluster_Out"=w572:T10)
        n266 = Unbundle By Name(w572) -> ("Car position slider Ref"=w576:refnum<vi>, "Info_for_driver Ref"=w574:refnum<vi>, "Car wash indicators Ref"=w573:refnum<vi>)
        n267 = property class="Slide (strict)"(reference=w576) -> ("Value"=w575:i8)  [unwired: 1 in, 2 out]
        n268 = case shown="6" w575 {
          tunnel: w574 -> [w581 _]
          tunnel: [w582 "Idle\nProgress: Timer \nProgress: Option6\n " ("State(s) in Front (\"\")")] -> w570
          tunnel: w573 -> [w580 w599]
          frame 0, Default {
            n269 = global read "Bad_position.vi" "Boolean"() -> (w583:bool)
            n270 = case shown="False" w583 {
              tunnel: w581 -> [w587 _]
              tunnel: ["Idle\nProgress: Option6" ("State(s) in Front (\"\")") "Idle\nProgress: Option6" ("State(s) in Front (\"\")")] -> w582
              tunnel: w580 -> [w584 _]
              frame False {
                n271 = property class="Clust"(reference=w584) -> ("Controls[]"=w585:refnum<vi>[])  [unwired: 1 in, 2 out]
                n272 = Index Array(array=w585, index #1=6 ("index"), index #2=8 ("index")) -> (element #1=w591:refnum<vi>, element #2=w589:refnum<vi>)
                n273 = property class="Str"(reference=w587, "Value"="JedŸ do stacji 3") -> ()  [unwired: 1 in, 2 out]
                n274 = global write "Bad_position.vi" "Boolean"(TRUE ("Boolean")) -> ()
                n275 = To Variant(anything=FALSE) -> (Variant=w592:variant)
                n276 = To Variant(anything=TRUE) -> (Variant=w596:variant)
                n277 = property class="Ctl"(reference=w591, "Value"=w592) -> ()  [unwired: 1 in, 2 out]
                n278 = property class="Ctl"(reference=w589, "Value"=w596) -> ()  [unwired: 1 in, 2 out]
              }
              frame True {
              }
            }
          }
          frame 6 {
            n279 = property class="Clust"(reference=w599) -> ("Controls[]"=w600:refnum<vi>[])  [unwired: 1 in, 2 out]
            n280 = Index Array(array=w600, index #1=6 ("index"), index #2=8 ("index")) -> (element #1=w606:refnum<vi>, element #2=w602:refnum<vi>)
            n281 = To Variant(anything=TRUE) -> (Variant=w605:variant)
            n282 = To Variant(anything=FALSE) -> (Variant=w609:variant)
            n283 = property class="Ctl"(reference=w606, "Value"=w605) -> ()  [unwired: 1 in, 2 out]
            n284 = property class="Ctl"(reference=w602, "Value"=w609) -> ()  [unwired: 1 in, 2 out]
          }
        }
        n285 = call <vilib>:"Add State(s) to Queue__JKI_lib_State_Machine.vi"("State(s) in Front (\"\")"=w570, "State(s) in (\"\")"=w579) -> ("States Out"=w578:string)  [unwired: 13 in]
      }
      frame "Progress: Option7" {
        # "Your code here.\n(You can make a copy of, or modify, this frame)"
        n286 = Unbundle By Name(w611) -> ("UI_Cluster_Out"=w612:T10)
        n287 = Unbundle By Name(w612) -> ("Car position slider Ref"=w616:refnum<vi>, "Info_for_driver Ref"=w614:refnum<vi>, "Car wash indicators Ref"=w613:refnum<vi>)
        n288 = property class="Slide (strict)"(reference=w616) -> ("Value"=w615:i8)  [unwired: 1 in, 2 out]
        n289 = case shown="0, Default" w615 {
          tunnel: w614 -> [w621 _]
          tunnel: [w622 "Idle\nProgress: Timer \nProgress: Option7\n " ("State(s) in Front (\"\")")] -> w610
          tunnel: w613 -> [w620 w639]
          frame 0, Default {
            n290 = global read "Bad_position.vi" "Boolean"() -> (w623:bool)
            n291 = case shown="False" w623 {
              tunnel: w621 -> [w627 _]
              tunnel: ["Idle\nProgress: Option7" ("State(s) in Front (\"\")") "Idle\nProgress: Option7" ("State(s) in Front (\"\")")] -> w622
              tunnel: w620 -> [w624 _]
              frame False {
                n292 = property class="Clust"(reference=w624) -> ("Controls[]"=w625:refnum<vi>[])  [unwired: 1 in, 2 out]
                n293 = Index Array(array=w625, index #1=7 ("index"), index #2=8 ("index")) -> (element #1=w631:refnum<vi>, element #2=w629:refnum<vi>)
                n294 = property class="Str"(reference=w627, "Value"="JedŸ do stacji 3") -> ()  [unwired: 1 in, 2 out]
                n295 = global write "Bad_position.vi" "Boolean"(TRUE ("Boolean")) -> ()
                n296 = To Variant(anything=FALSE) -> (Variant=w632:variant)
                n297 = To Variant(anything=TRUE) -> (Variant=w636:variant)
                n298 = property class="Ctl"(reference=w631, "Value"=w632) -> ()  [unwired: 1 in, 2 out]
                n299 = property class="Ctl"(reference=w629, "Value"=w636) -> ()  [unwired: 1 in, 2 out]
              }
              frame True {
              }
            }
          }
          frame 6 {
            n300 = property class="Clust"(reference=w639) -> ("Controls[]"=w640:refnum<vi>[])  [unwired: 1 in, 2 out]
            n301 = Index Array(array=w640, index #1=7 ("index"), index #2=8 ("index")) -> (element #1=w646:refnum<vi>, element #2=w642:refnum<vi>)
            n302 = To Variant(anything=TRUE) -> (Variant=w645:variant)
            n303 = To Variant(anything=FALSE) -> (Variant=w649:variant)
            n304 = property class="Ctl"(reference=w646, "Value"=w645) -> ()  [unwired: 1 in, 2 out]
            n305 = property class="Ctl"(reference=w642, "Value"=w649) -> ()  [unwired: 1 in, 2 out]
          }
        }
        n306 = call <vilib>:"Add State(s) to Queue__JKI_lib_State_Machine.vi"("State(s) in Front (\"\")"=w610, "State(s) in (\"\")"=w619) -> ("States Out"=w618:string)  [unwired: 13 in]
      }
      frame "Progress: Reset variables_to leave" {
        # "Your code here.\n(You can make a copy of, or modify, this frame)"
        n307 = Unbundle By Name(w655) -> ("UI_Cluster_Out.Car wash indicators Ref"=w654:refnum<vi>, "UI_Cluster_Out.Info_for_driver Ref"=w651:refnum<vi>)
        n308 = property class="Str"(reference=w651, "Value"="JedŸ do wyjazdu") -> ()  [unwired: 1 in, 2 out]
        n309 = property class="Clust"(reference=w654, "Value"=T2 {"Under Body Wash"=FALSE, "Bug remover"=FALSE, "Pre-soak"=FALSE, "High pressure Wash"=FALSE, "Low pressure Wax"=FALSE, "Spot free Rinse "=FALSE, "Tire Shine Foam "=FALSE, "Air Dry "=FALSE, "Vehicle Out of Position"=TRUE} ("Car wash indicators")) -> ()  [unwired: 1 in, 2 out]
        n310 = call <vilib>:"Add State(s) to Queue__JKI_lib_State_Machine.vi"("State(s) in Front (\"\")"="Database: Add to Base" ("State(s) in Front (\"\")"), "State(s) in (\"\")"=w658) -> ("States Out"=w657:string)  [unwired: 13 in]
      }
      frame "Progress: Wait for slider" {
        # "Your code here.\n(You can make a copy of, or modify, this frame)"
        n311 = case shown="7" "Car position slider" {
          tunnel: ["Idle\n Progress: Wait for slider " ("State(s) in Front (\"\")") _] -> w660
          frame 0, Default {
          }
          frame 7 {
            w667 = i8 0 items=["Entry", "|", "Station 1", "||", "Station 2", "|||", "Station 3", "Exit"] ("Car position slider")
            n312 = Wait (ms)(milliseconds to wait=u32 200) -> ()  [unwired: 1 out]
            n313 = local write "Car position slider"(w667) -> ()
            n314 = property on="Car position slider" class="Slide (strict)"("DisabledEnum"=T9."Disabled" ("Disabled")) -> ()  [unwired: 2 in, 2 out]
          }
        }
        n315 = call <vilib>:"Add State(s) to Queue__JKI_lib_State_Machine.vi"("State(s) in Front (\"\")"=w660, "State(s) in (\"\")"=w664) -> ("States Out"=w663:string)  [unwired: 13 in]
      }
      frame "---------- Database ----------" {
        n316 = call <vilib>:"Add State(s) to Queue__JKI_lib_State_Machine.vi"("State(s) in (\"\")"=w671) -> ("States Out"=w670:string)  [unwired: 14 in]
      }
      frame "Database: Add to Base" {
        n317 = local read "License Plate"() -> (w673:string)
        n318 = local read "Array"() -> (w682:i8[])
        n319 = call "Array2String.vi"("Plate"=w673, "Array_Input"=w682) -> ("String_Out"=w678:string)  [unwired: 9 in]
        "SQL_Expression" <- w678
        n320 = call-poly <vilib>:"Open.vi"("db file"=path "carwash.db") -> ("error out"=w675:errorcluster, "SQLite Connection"=w679:refnum<class "Connection.lvclass">)  [unwired: 9 in]
        n321 = call-poly <vilib>:"Execute SQL (Poly).vi"("error in (no error)"=w675, "SQL"=w678, "SQLite Connection in"=w679) -> ("error out"=w676:errorcluster, "SQLite Connection"=w677:refnum<class "Connection.lvclass">)  [unwired: 5 in, 2 out]
        n322 = call-dynamic "Close.vi"("error in (no error)"=w676, "SQLite Connection in"=w677) -> ()  [unwired: 9 in, 1 out]
        n323 = call <vilib>:"Add State(s) to Queue__JKI_lib_State_Machine.vi"("State(s) in (\"\")"=w684) -> ("States Out"=w683:string)  [unwired: 14 in]
      }
      frame "Database: Show database" {
        n324 = local read "Show Database"() -> (w685:bool)
        n325 = case shown="True" w685 {
          frame False {
          }
          frame True {
            n326 = call-poly <vilib>:"Open.vi"("db file"=path "carwash.db") -> ("error out"=w692:errorcluster, "SQLite Connection"=w695:refnum<class "Connection.lvclass">)  [unwired: 9 in]
            n327 = call-poly <vilib>:"Execute SQL (Poly).vi"("error in (no error)"=w692, "SQL"="SELECT * FROM Plates_Options", "SQLite Connection in"=w695) -> ("error out"=w693:errorcluster, "Result Set"=→"Result Set":string[][], "SQLite Connection"=w694:refnum<class "Connection.lvclass">)  [unwired: 5 in, 1 out]
            n328 = call-dynamic "Close.vi"("error in (no error)"=w693, "SQLite Connection in"=w694) -> ()  [unwired: 9 in, 1 out]
          }
        }
        n329 = call <vilib>:"Add State(s) to Queue__JKI_lib_State_Machine.vi"("State(s) in (\"\")"=w689) -> ("States Out"=w688:string)  [unwired: 14 in]
      }
    }
  }
  n330 = call "IMAQ OCR Read Character Set File"("File Path"=path "letter.abc", "error in (no error)"=w16, "IMAQ OCR Session"=w15) -> ("error out"=w4:errorcluster, "IMAQ OCR Session (dup)"=w18:T6)  [unwired: 6 in, 1 out]
  n331 = call "IMAQ Create"("Image Name"="untitled") -> ("New Image"=w12:T1)  [unwired: 4 in, 1 out]
  n332 = call <vilib>:"IMAQdx Configure Grab.vi"("error in"=w7, "Session In"=w8) -> ("error out"=w10:errorcluster, "Session Out"=w9:T5)  [unwired: 8 in]
  n333 = call "IMAQ Convert Rectangle to ROI"("Rectangle"=T4 {"Left"=271, "Top"=350, "Right"=1687, "Bottom"=657, "Rotation"=0.0}) -> ("ROI Descriptor"=w19:T13)  [unwired: 8 in, 1 out]
  n334 = while {
    tunnel: w10 -> [w708]
    tunnel: w12 -> [w707]
    shift-right: [w699] -> w13
    shift-left: w9 -> [w709]
    tunnel: w18 -> [w706]
    tunnel: w19 -> [w705]
    shift-right: [w701] -> _
    shift-left: FALSE -> [w703]
    tunnel: [w700] -> w5
    tunnel: [w697] -> w2
    stop <- w698 stop-if-true
    n335 = case shown="False" w703 {
      tunnel: w709 -> [w730 w734]
      tunnel: w708 -> [w729 w733]
      tunnel: w707 -> [w728 _]
      tunnel: [w727 w734] -> w699
      tunnel: [w723 _] -> w700
      tunnel: w706 -> [w719 _]
      tunnel: w705 -> [w717 _]
      tunnel: [w715 w733] -> w697
      tunnel: [w714 w732] -> w704
      tunnel: [w713 w731] -> w702
      frame False {
        n336 = call <vilib>:"IMAQdx Grab2.vi"("error in"=w729, "Image In"=w728, "Session In"=w730) -> ("error out"=w721:errorcluster, "Image Out"=w723:T1, "Session Out"=w727:T5)  [unwired: 5 in, 1 out]
        n337 = call "IMAQ Clear Overlay"("error in (no error)"=w721, "Image"=w723) -> ("error out"=w720:errorcluster, "Image Out"=w722:T1)  [unwired: 8 in]
        n338 = call "IMAQ OCR Read Text 4"("IMAQ OCR Session"=w719, "ROI Descriptor"=w717, "Image"=w722, "error in (no error)"=w720) -> ("Image (dup)"=w726:T1, "Read String"=w714:string, "ROI Bounding Characters"=w724:T14, "error out"=w718:errorcluster)  [unwired: 5 in, 3 out]
        "Read String" <- w714
        n339 = call "IMAQ Overlay ROI"("Colors (Green)"=u32[] [16723200], "error in (no error)"=w718, "ROI Descriptor"=w724, "Image"=w726) -> ("error out"=w715:errorcluster, "Image Out"=→"Image":T1)  [unwired: 6 in]
        n340 = local read "Start Button"() -> (w713:bool)
      }
      frame True {
        n341 = local read "Start Button"() -> (w731:bool)
        n342 = local read "License Plate"() -> (w732:string)
      }
    }
    n343 = case shown="True" w702 {
      selector: w702 -> [w710 w711]
      tunnel: w704 -> [_ w712]
      tunnel: [w710 w711] -> w701
      frame False {
      }
      frame True {
        n344 = local write "License Plate"(w712) -> ()
      }
    }
    n345 = local read "Exit_Panel"() -> (w698:bool)
  }
  n346 = disable-structure shown="Disabled" {
    frame Disabled {
      n347 = call-poly <vilib>:"Open.vi"("db file"=path "carwash.db") -> ()  [unwired: 9 in, 2 out]
      n348 = call-poly <vilib>:"Execute SQL (Poly).vi"() -> ()  [unwired: 10 in, 2 out]
      n349 = call-dynamic "Close.vi"() -> ()  [unwired: 11 in, 1 out]
    }
    frame Enabled {
    }
  }
  n350 = disable-structure shown="Enabled" {
    disable-tunnel: w5 -> [w736 _]
    frame Disabled {
      n351 = call "Vision Assistant"("Image In"=w736) -> ()  [unwired: 25 in, 2 out]
    }
    frame Enabled {
    }
  }
  n352 = call <vilib>:"IMAQdx Close Camera.vi"("error in"=w2, "Session In"=w13) -> ("error out"=w1:errorcluster)  [unwired: 9 in]
  n353 = call <vilib>:"Simple Error Handler.vi"("error in (no error)"=w1) -> ()  [unwired: 4 in, 5 out]
